vi "browser.vi"(3 "?":refnum<k7>(container), 10 "stop":bool, 11 "browser_link":path) -> ()   [LabVIEW 2017]
panel:
  out "Path":path
  in  "OK Button":bool
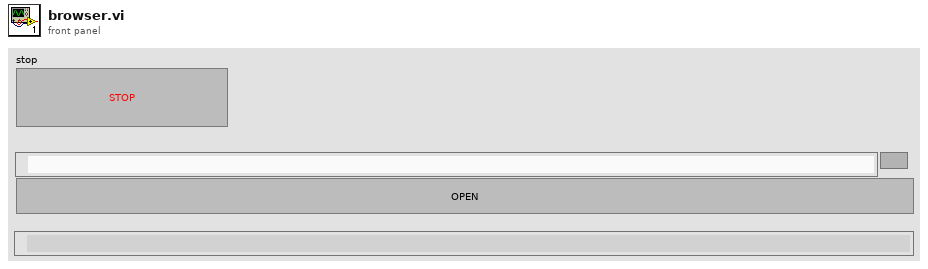
[diagram p1: front panel]
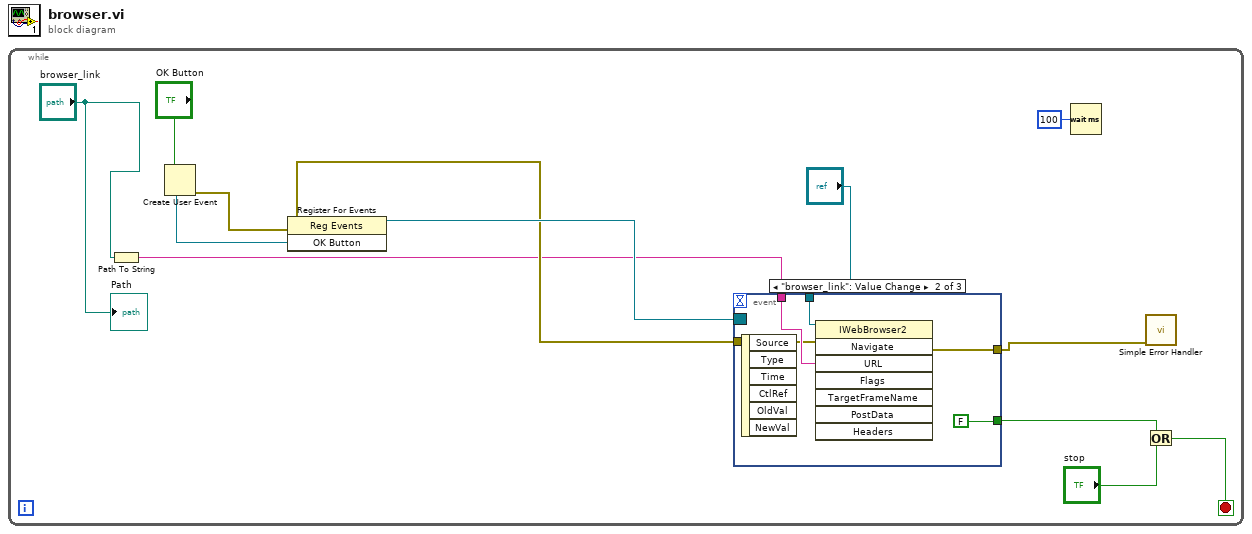
[diagram p0: block diagram]
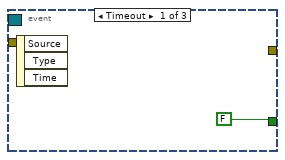
[diagram p2: hidden frame]
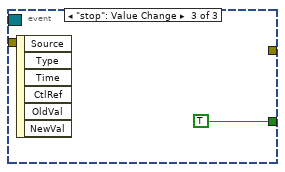
[diagram p3: hidden frame]
diagram:
  n1 = while {
    stop <- w4 stop-if-true
    n2 = Path To String(path="browser_link") -> (string=w9:string)
    n3 = Create User Event(user event datatype="OK Button") -> (user event=w8:refnum<user-event>, error out=w7:errorcluster)  [unwired: 1 in]
    n4 = register-events(error in=w7, w8) -> (reference out=w13:refnum<event-registration>, error out=w12:errorcluster)  [unwired: 1 in]
    n5 = event shown="[1] \"browser_link\": Value Change" {
      selector: w13 -> [_ _ _]
      dyn-events: _ -> [_ _ _]
      timeout: _ -> [_ _ _]
      tunnel: "?" -> [_ w18 _]
      tunnel: w9 -> [_ w17 _]
      tunnel: [_ w16 _] -> w11
      tunnel: w12 -> [_ w16 _]
      tunnel: [FALSE FALSE TRUE] -> w6
      event Timeout {
        n6 = event-data() -> ()  [unwired: 1 in, 3 out]
      }
      event "browser_link": Value Change {
        n7 = event-data() -> ()  [unwired: 1 in, 6 out]
        n8 = invoke class="IWebBrowser2" method="Navigate"(reference=w18, "URL"=w17) -> ()  [unwired: 6 in, 8 out]
      }
      event "stop": Value Change {
        n9 = event-data() -> ()  [unwired: 1 in, 6 out]
      }
    }
    n10 = Wait (ms)(milliseconds to wait=u32 100) -> ()  [unwired: 1 out]
    n11 = call <vilib>:"Simple Error Handler.vi"("error in (no error)"=w11) -> ()  [unwired: 4 in, 5 out]
    n12 = Or(x=w6, y="stop") -> (x .or. y?=w4:bool)
    "Path" <- "browser_link"
  }
